vi "CountZero.vi"(8 "error in (no error)":errorcluster, 11 "SimpleAF in":refnum<class "Counter.lvclass">) -> (0 "error out":errorcluster, 3 "SimpleAF out":refnum<class "Counter.lvclass">)   [LabVIEW 2013, in "Counter.lvclass"]
uses:
  Counter.lvclass
  Counter.lvclass/Counter.ctl
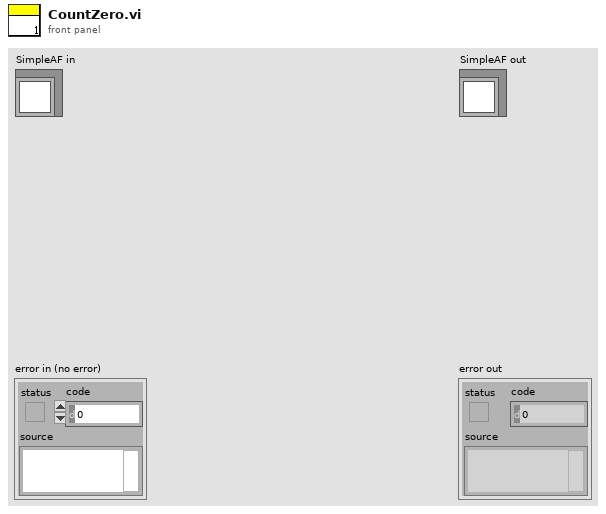
[diagram p1: front panel]
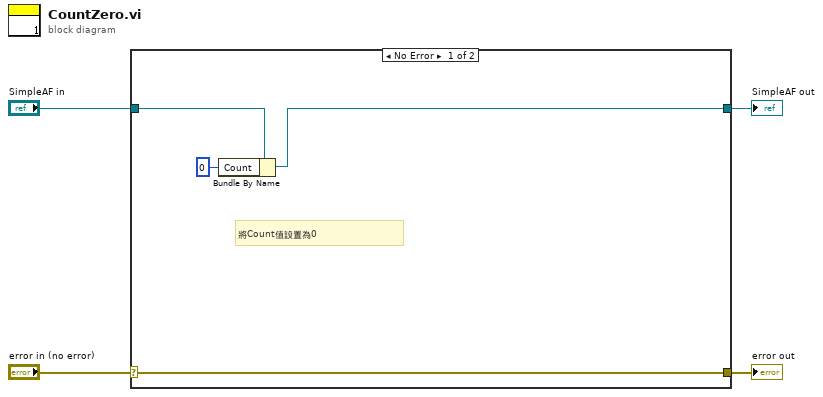
[diagram p0: block diagram]
diagram:
  n1 = case shown="No Error" "error in (no error)" {
    selector: "error in (no error)" -> [w8 w10]
    tunnel: [w8 w10] -> w3
    tunnel: [w5 w9] -> w1
    tunnel: "SimpleAF in" -> [w6 w9]
    frame No Error {
      # "將Count值設置為0"
      n2 = Bundle By Name(cluster=w6, "Count"=0) -> (w5:refnum<class "Counter.lvclass">)
    }
    frame Error {
    }
  }
  "error out" <- w3
  "SimpleAF out" <- w1
